vi "chart series set error bars endcap.vi"(8 "error in (no error)":errorcluster, 10 "endcap":u8, 11 "error_bars":u32) -> (0 "error out":errorcluster)   [LabVIEW 8.6]
doc: "void chart_series_set_error_bars_endcap(lxw_series_error_bars error_bars, uint8_t endcap);"
uses:
  pending_lvxlsxwriter/xlsxwriter.dll
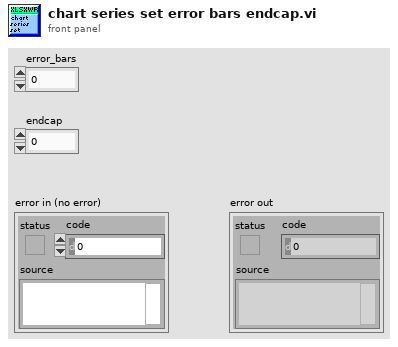
[diagram p1: front panel]
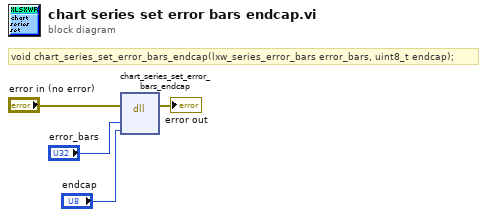
[diagram p0: block diagram]
diagram:
  # "void chart_series_set_error_bars_endcap(lxw_series_error_bars error_bars, uint8_t endcap);"
  n1 = dll-call lib="C:/Users/WDAGUtilityAccount/Desktop/pending_lvxlsxwriter/xlsxwriter.*" fn="chart_series_set_error_bars_endcap"(error in="error in (no error)", "error_bars"="error_bars", "endcap"="endcap") -> (error out=→"error out":errorcluster)  [unwired: 5 in, 1 out]
